vi "FPGAController_v4.vi"() -> ()   [LabVIEW 2013]
uses:
  <vilib>/rvi/interface/nirviOpenFPGA/nirviOpenFPGA.xnode
  <vilib>/rvi/interface/nirviMethod/nirviMethod.xnode
  <vilib>/rvi/interface/nirviReadWriteControl/nirviReadWriteControl.xnode
  <vilib>/rvi/interface/nirviCloseFPGA/nirviCloseFPGA.xnode
  <vilib>/addons/database/NI_Database_API.lvlib
  <vilib>/addons/database/Recordset.llb/Rec Fetch Recordset Data (R).vi
  <vilib>/addons/database/Connection.llb/Conn Execute.vi
  <vilib>/addons/database/_DB Variant To Data/Database Variant To Data.xnode
  <vilib>/addons/database/Recordset.llb/Rec Destroy - Connection.vi
  <vilib>/Utility/miscctls.llb/LVPointTypeDef.ctl
  <userlib>/Accelerator/User Interface/Executables/FPGAController_v4/data/correlationwithf_FPGATarget_FPGAcode60214_dpdmgs7o1BA.lvbitx
  <userlib>/_OpenG.lib/file/file.llb/Strip Path Extension - Path__ogtk.vi
  <userlib>/_OpenG.lib/comparison/comparison.llb/Boolean Changed__ogtk.vi
  <userlib>/_OpenG.lib/comparison/comparison.llb/DBL Changed__ogtk.vi
  <vilib>/rvi/errors/niLvFpgaMergeErrorWithErrorCode.vi
  <vilib>/FPGAPlugInAG/PXI-7954R/niLvFpga_Open_PXI-7954R.vi
panel:
  out "Time Betwee Shots":dbl
  out "Del Armed":bool
  in  "Lower Threshold":bool
  in  "Raise Threshold":bool
  out "Update Threshold":bool
  in  "Min. Time\nBetween Shots (s)":dbl
  in  "Rate Limiting":bool
  out "Armed":bool
  in  "Add Delay":bool
  in  "Delay Name":string
  in  "Delay Value":dbl=3.0 min=0.0
  in  "Delay Ring":dbl(ring)=3.15039 items=["Ablation Chamber"=6.45, "LEIL Chamber"=4.318, "Thid Detector"=3.15039, "Custom"=0.0]
  in  "Rearm Trigger":bool
  in  "One Shot Mode":bool
  out "Last Update:":timestamp
  out "Updating FPGA":bool
  out "Sensitivity":dbl
  out "error out":errorcluster
  out "Low Mass Limit":fxp<+,31,17>
  out "High Mass Limit":fxp<+,31,17>
  out "stopping":bool
  in  "Auto Threshold":bool
  out "Peletron (MV)":dbl=2.0
  out "High Mass (kg)":dbl=inf
  out "Low Mass (kg)":dbl
  out "High Charge Limit":i16
  out "Low Charge Limit":i16
  out "High velocity count":i32=210
  out "Low velocity count":i32=21000
  in  "stop":bool
  in  "Peak-Threshold Factor":dbl=2.0
  out "Low Charge Limit (fC)":dbl
  out "High Charge Limit (fC)":dbl=100.0
  out "High Velocity":dbl=100000.0
  out "Low Velocity":dbl=1000.0
  out "Filter 7 Peak":i32=7483
  out "Filter 6 Peak":i32=9863
  out "Filter 5 Peak":i32=13910
  out "Filter 4 Peak":i32=18191
  out "Filter 3 Peak":i32=46254
  out "Filter 2 Peak":i32=120664
  out "Filter 1 Peak":i32=295996
  in  "Filter7 Threshold":i32=-21165
  in  "Filter6 Threshold":i32=-29358
  in  "Filter5 Threshold":i32=-41730
  in  "Filter4 Threshold":i32=-54306
  in  "Filter3 Threshold":i32=-138762
  in  "Filter2 Threshold":i32=-361992
  in  "Filter1 Threshold":i32=-887988
  in  "Zero Peak Values":bool
  in  "Assign Threshold":bool
  in  "Run Mode":bool
  # "Settings"
  # "Dubugging"
  # "Independent Variable"
  # "Low Vel."
  # "High Vel."
  # "Low Q (fC)"
  # "High Q (fC)"
  # "Plate Control While Loop Counter"
  # "Low Mass (kg)"
  # "High Mass (kg)"
  # "Sens. (V/pC)"
  # "Peletron (MV)"
  # "Current Value of Running Average"
  # "Peak Threshold Factor"
  # "Delay Trigger"
  # "Dist. from 2nd Det. (m)"
  # "Name"
  # "Peak Values"
  # "Peak 1"
  # "Peak 2"
  # "Peak 3"
  # "Peak 4"
  # "Peak 5"
  # "Peak 6"
  # "Peak 7"
  # "Thresholds"
  # "Threshold 1"
  # "Threshold 2"
  # "Threshold 3"
  # "Threshold 4"
  # "Threshold 5"
  # "Threshold 6"
  # "Threshold 7"
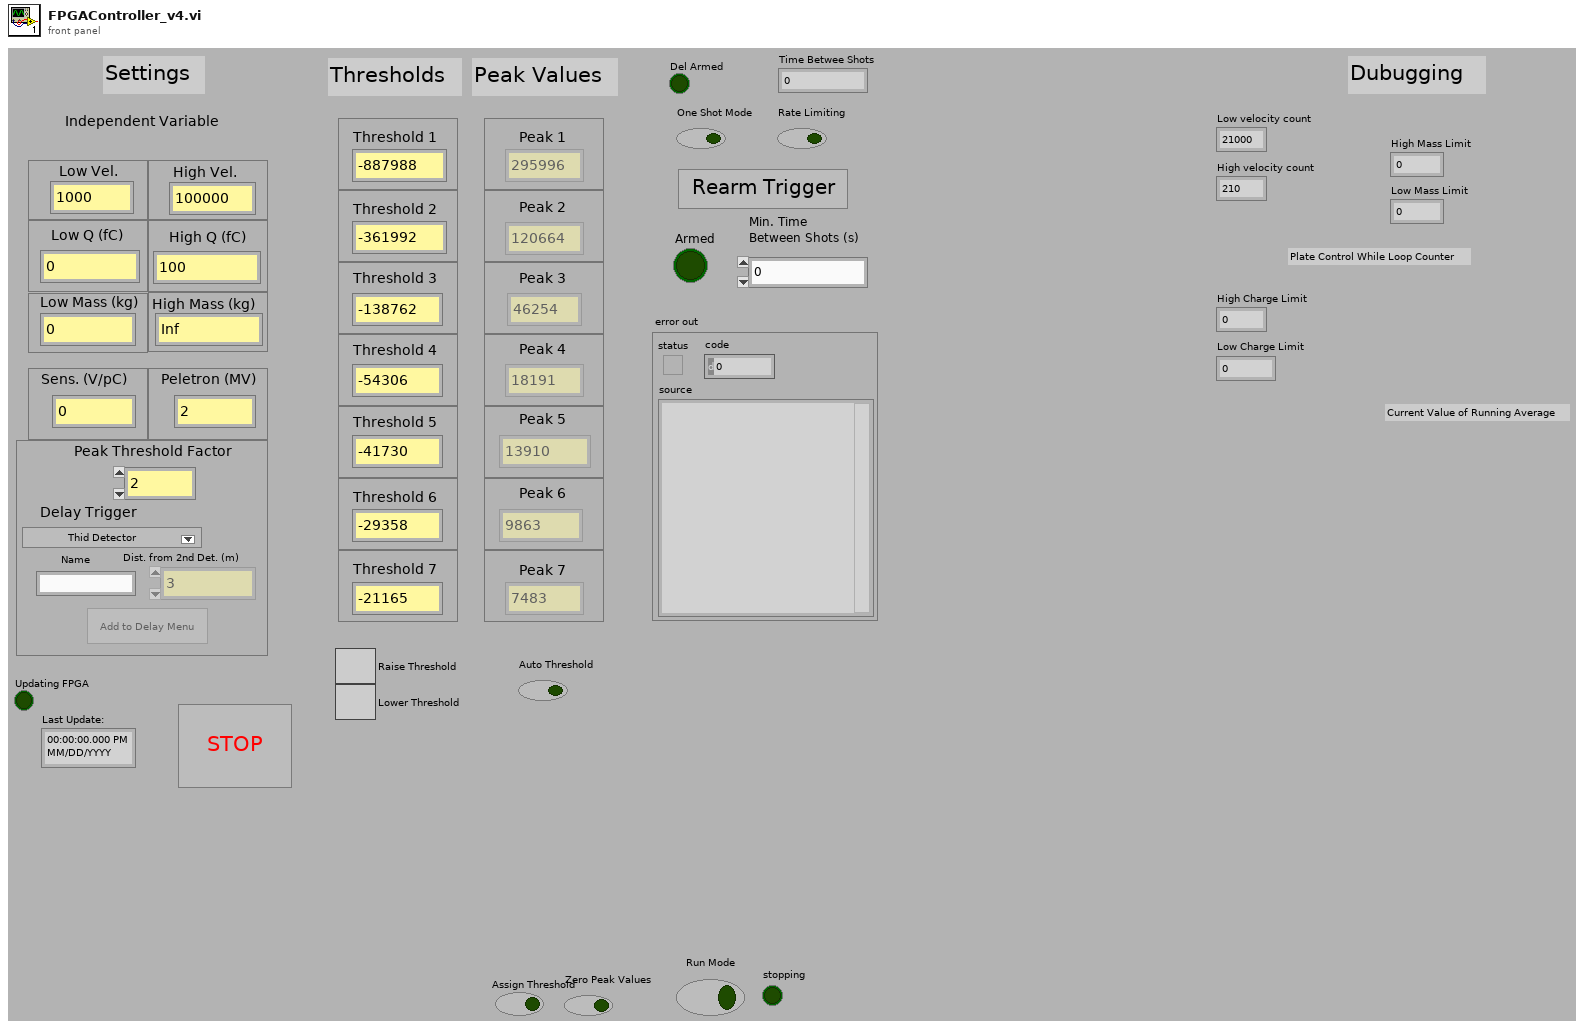
[diagram p1: front panel]
types:
  T1 = typedef "LVPointTypeDef.ctl" = cluster{"Horizontal":i16, "Vertical":i16}
  T2 = enum8{"Enabled", "Disabled", "Disabled and Grayed Out"}
  T3 = typedef "NI_Database_API.lvlib/Conn ObjectReference.ctl" = refnum<k1>
  T4 = cluster{"Filter 1 Peak":i32, "Filter 2 Peak":i32, "Filter 3 Peak":i32, "Filter 4 Peak":i32, "Filter 5 Peak":i32, "Filter 6 Peak":i32, "Filter 7 Peak":i32}
  T5 = typedef "NI_Database_API.lvlib/Rec ObjectReference.ctl" = refnum<k1>
  T6 = typedef "LVStringsAndValuesArrayTypeDef_DBL.ctl" = cluster{"String":string, "Value":dbl}[]
  T7 = cluster{"Numeric":dbl, "Numeric":dbl, "Numeric":dbl, "Numeric":dbl, "Numeric":dbl, "Numeric":dbl, dbl, dbl, "Value":dbl, fxp<+,16,7>, bool}
  T8 = cluster{"Low Velocity Count":i32, "High Velocity Count":i32, "Low Charge Limit (ADC ticks)":i16, "High Charge Limit (ADC ticks)":i16, "Low Mass (ADC*cycle^2)":i64, "High Mass (ADC*cycle^2)":i64, "Mult":fxp<+,16,7>, "Mult Use?":bool}
  T9 = cluster{"Filter 1 Detector 3 Correlation":void, "Filter 2 Detector 3 Correlation":void, "Filter 3 Detector 3 Correlation":void, "Filter 4 Detector 3 Correlation":void, "Filter 5 Detector 3 Correlation":void, "Filter 6 Detector 3 Correlation":void, "Filter 7 Detector 3 Correlation":void}
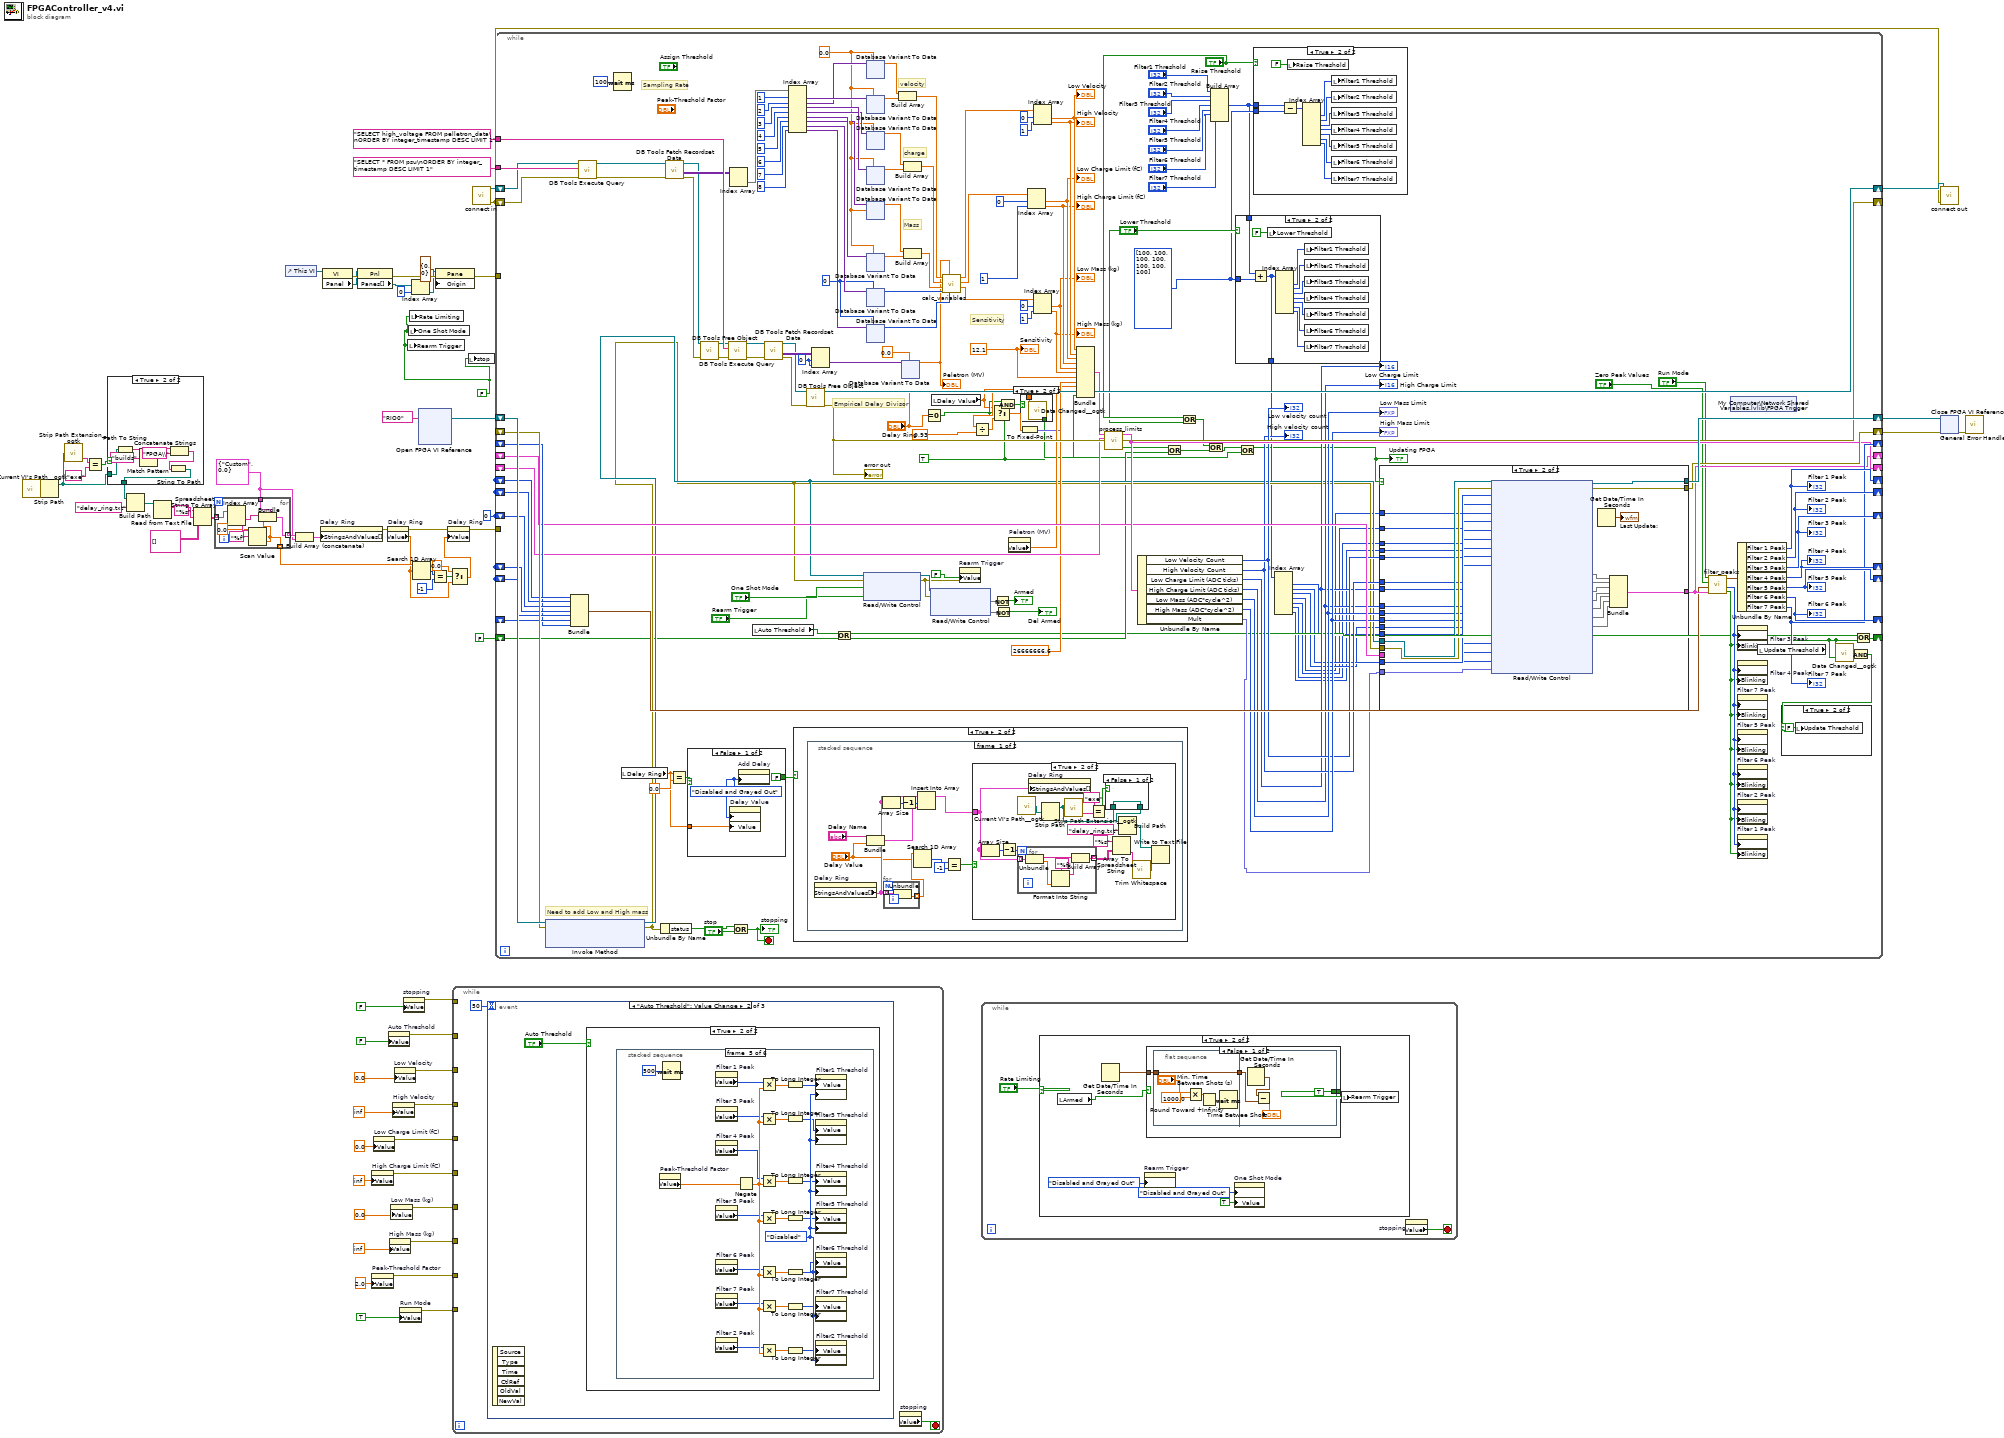
[diagram p0: block diagram]
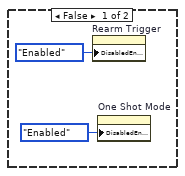
[diagram p3: hidden frame]
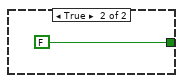
[diagram p4: hidden frame]
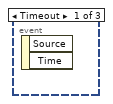
[diagram p5: hidden frame]
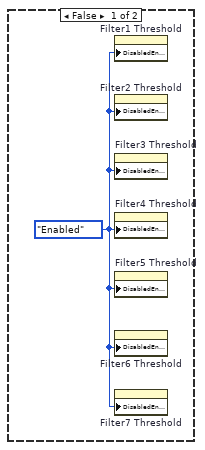
[diagram p6: hidden frame]
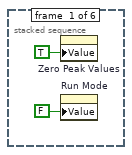
[diagram p7: hidden frame]
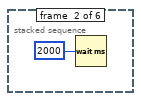
[diagram p8: hidden frame]
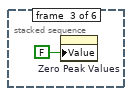
[diagram p9: hidden frame]
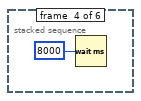
[diagram p10: hidden frame]
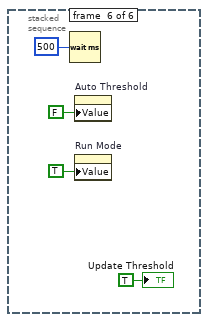
[diagram p11: hidden frame]
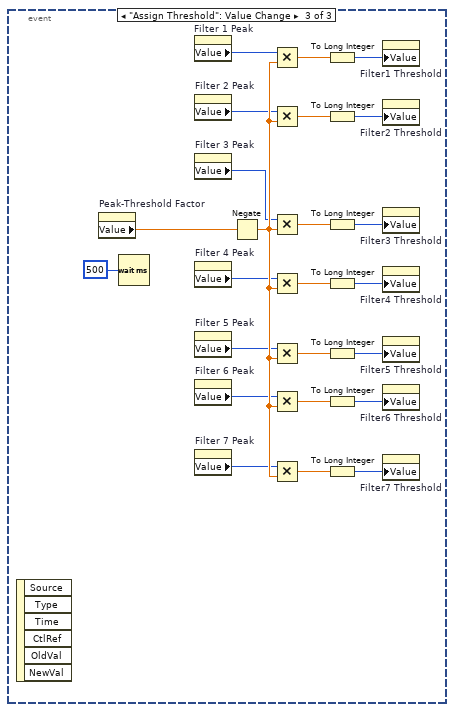
[diagram p12: hidden frame]
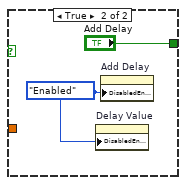
[diagram p17: hidden frame]
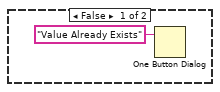
[diagram p19: hidden frame]
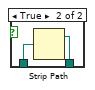
[diagram p20: hidden frame]
diagram:
  w17 = cluster{"String":string, "Value":dbl} {"String"="Custom", "Value"=0.0}
  w27 = FALSE
  w66 = 0
  n1 = call <userlib>:"Current VI's Path__ogtk.vi"() -> ("Current VI's Path (+ Relative)"=w26:path)  [unwired: 1 in]
  n2 = Strip Path(path=w26) -> (stripped path=w12:path)  [unwired: 1 out]
  n3 = call-poly <userlib>:"Strip Path Extension__ogtk.vi"("path"=w12) -> ("extension"=w16:string)  [unwired: 1 out]
  n4 = Equal?(x=w16, y="exe") -> (x = y?=w13:bool)
  n5 = case shown="True" w13 {
    tunnel: w12 -> [w68 w75]
    tunnel: [w68 w69] -> w11
    frame False {
    }
    frame True {
      n6 = Path To String(path=w75) -> (string=w74:string)
      n7 = Match Pattern(string=w74, regular expression="builds") -> (before substring=w72:string)  [unwired: 1 in, 3 out]
      n8 = Concatenate Strings(w72, "FPGA\\" ("string")) -> (w70:string)
      n9 = String To Path(string=w70) -> (path=w69:path)
    }
  }
  n10 = Build Path(base path=w11, name or relative path="delay_ring.txt") -> (appended path=w14:path)
  n11 = Read from Text File(file (use dialog)=w14) -> (text=w24:string)  [unwired: 3 in, 3 out]
  n12 = Spreadsheet String To Array(format string="%s", spreadsheet string=w24, array type (2D Dbl)=string[][] []) -> (array=w21:string[][])  [unwired: 1 in]
  n13 = for {
    tunnel: w21 -> [w83] mode=indexing
    tunnel: w17 -> [w81]
    tunnel: [w77] -> w18 mode=indexing
    tunnel: [w76] -> w10 mode=indexing
    n14 = Index Array(array=w83) -> (element #1=w82:string, element #2=w80:string)  [unwired: 2 in]
    n15 = Scan Value(string=w80, format string="%f", default (0 dbl)=0.0) -> (value=w76:dbl)  [unwired: 1 out]
    n16 = Bundle(cluster=w81, "String"=w82, "Value"=w76) -> (w77:cluster{"String":string, "Value":dbl})
  }
  n17 = control-ref of="This VI"() -> (w38:refnum<vi>)
  n18 = Build Array (concatenate)(w18, w17) -> (w20:cluster{"String":string, "Value":dbl}[])
  n19 = property on="Delay Ring" class="Ring (strict)"("StringsAndValues[]"=w20) -> (error out=w19:errorcluster)  [unwired: 2 in, 1 out]
  n20 = property class="VI"(reference=w38) -> (error out=w37:errorcluster, "Panel"=w36:refnum<vi>)  [unwired: 1 in, 1 out]
  n21 = property class="Pnl"(reference=w36, error in=w37) -> (error out=w35:errorcluster, "Panes[]"=w34:refnum<vi>[])  [unwired: 1 out]
  n22 = property on="High Charge Limit (fC)" class="DigNum (strict)"("Value"=inf ("High Charge Limit (fC)")) -> (error out=w53:errorcluster)  [unwired: 2 in, 1 out]
  n23 = property on="Peak-Threshold Factor" class="DigNum (strict)"("Value"=2.0 ("Peak-Threshold Factor")) -> (error out=w47:errorcluster)  [unwired: 2 in, 1 out]
  n24 = property on="Low Charge Limit (fC)" class="DigNum (strict)"("Value"=0.0 ("Low Charge Limit (fC)")) -> (error out=w55:errorcluster)  [unwired: 2 in, 1 out]
  n25 = property on="Delay Ring" class="Ring (strict)"(error in=w19) -> (error out=w9:errorcluster, "Value"=w3:dbl)  [unwired: 1 in, 1 out]
  n26 = property on="Auto Threshold" class="Bool (strict)"("Value"=FALSE ("Auto Threshold")) -> (error out=w61:errorcluster)  [unwired: 2 in, 1 out]
  n27 = property on="High Mass (kg)" class="DigNum (strict)"("Value"=inf ("High Mass (kg)")) -> (error out=w49:errorcluster)  [unwired: 2 in, 1 out]
  n28 = property on="Low Mass (kg)" class="DigNum (strict)"("Value"=0.0 ("Low Mass (kg)")) -> (error out=w51:errorcluster)  [unwired: 2 in, 1 out]
  n29 = property on="High Velocity" class="DigNum (strict)"("Value"=inf ("High Velocity")) -> (error out=w57:errorcluster)  [unwired: 2 in, 1 out]
  n30 = property on="Low Velocity" class="DigNum (strict)"("Value"=0.0 ("Low Velocity")) -> (error out=w59:errorcluster)  [unwired: 2 in, 1 out]
  n31 = property on="Run Mode" class="Bool (strict)"("Value"=TRUE ("Run Mode")) -> (error out=w45:errorcluster)  [unwired: 2 in, 1 out]
  n32 = property on="stopping" class="Bool (strict)"("Value"=FALSE ("stopping")) -> (error out=w63:errorcluster)  [unwired: 2 in, 1 out]
  n33 = local write "Rearm Trigger"(w27) -> ()
  n34 = local write "One Shot Mode"(w27) -> ()
  n35 = local write "Rate Limiting"(w27) -> ()
  n36 = Index Array(array=w34, index=0) -> (element=w32:refnum<vi>)
  n37 = Search 1D Array(1D array=w10, element=w3) -> (index of element=w7:i32)  [unwired: 1 in]
  n38 = xnode "Open FPGA VI Reference"("resource name"=tag "RIO0") -> ("FPGA VI Reference Out"=w29:refnum<k20>)  [unwired: 1 in, 1 out]
  n39 = Equal?(x=w7, y=-1) -> (x = y?=w5:bool)
  n40 = property class="Pane"(reference=w32, error in=w35, "Origin"=T1 {"Horizontal"=0, "Vertical"=0}) -> (error out=w30:errorcluster)  [unwired: 1 out]
  n41 = Select(t=0.0, s=w5, f=w3) -> (s? t:f=w4:dbl)
  n42 = property on="Delay Ring" class="Ring (strict)"(error in=w9, "Value"=w4) -> (error out=w8:errorcluster)  [unwired: 1 in, 1 out]
  n43 = while {
    tunnel: w63 -> [_]
    tunnel: w61 -> [_]
    tunnel: w59 -> [_]
    tunnel: w57 -> [_]
    tunnel: w55 -> [_]
    tunnel: w53 -> [_]
    tunnel: w51 -> [_]
    tunnel: w49 -> [_]
    tunnel: w47 -> [_]
    tunnel: w45 -> [_]
    stop <- w85 stop-if-true
    n44 = event shown="[1] \"Auto Threshold\": Value Change" {
      selector: _ -> [_ _ _]
      dyn-events: _ -> [_ _ _]
      timeout: 50 -> [_ _ _]
      event Timeout {
        n45 = event-data() -> ()  [unwired: 1 in, 2 out]
      }
      event "Auto Threshold": Value Change {
        n46 = event-data() -> ()  [unwired: 1 in, 6 out]
        n47 = case shown="True" "Auto Threshold" {
          frame False {
            w87 = T2."Enabled" ("Disabled")
            n48 = property on="Filter1 Threshold" class="DigNum (strict)"("DisabledEnum"=w87) -> ()  [unwired: 2 in, 2 out]
            n49 = property on="Filter2 Threshold" class="DigNum (strict)"("DisabledEnum"=w87) -> ()  [unwired: 2 in, 2 out]
            n50 = property on="Filter3 Threshold" class="DigNum (strict)"("DisabledEnum"=w87) -> ()  [unwired: 2 in, 2 out]
            n51 = property on="Filter4 Threshold" class="DigNum (strict)"("DisabledEnum"=w87) -> ()  [unwired: 2 in, 2 out]
            n52 = property on="Filter5 Threshold" class="DigNum (strict)"("DisabledEnum"=w87) -> ()  [unwired: 2 in, 2 out]
            n53 = property on="Filter6 Threshold" class="DigNum (strict)"("DisabledEnum"=w87) -> ()  [unwired: 2 in, 2 out]
            n54 = property on="Filter7 Threshold" class="DigNum (strict)"("DisabledEnum"=w87) -> ()  [unwired: 2 in, 2 out]
          }
          frame True {
            n55 = stacked-sequence {
              frame #0 {
                n56 = property on="Zero Peak Values" class="Bool (strict)"("Value"=TRUE ("Zero Peak Values")) -> ()  [unwired: 2 in, 2 out]
                n57 = property on="Run Mode" class="Bool (strict)"("Value"=FALSE ("Run Mode")) -> ()  [unwired: 2 in, 2 out]
              }
              frame #1 {
                n58 = Wait (ms)(milliseconds to wait=u32 2000) -> ()  [unwired: 1 out]
              }
              frame #2 {
                n59 = property on="Zero Peak Values" class="Bool (strict)"("Value"=FALSE ("Zero Peak Values")) -> ()  [unwired: 2 in, 2 out]
              }
              frame #3 {
                n60 = Wait (ms)(milliseconds to wait=u32 8000) -> ()  [unwired: 1 out]
              }
              frame #4 {
                w117 = T2."Disabled" ("Disabled")
                n61 = property on="Peak-Threshold Factor" class="DigNum (strict)"() -> ("Value"=w102:dbl)  [unwired: 2 in, 2 out]
                n62 = Wait (ms)(milliseconds to wait=u32 500) -> ()  [unwired: 1 out]
                n63 = property on="Filter 1 Peak" class="DigNum (strict)"() -> ("Value"=w100:i32)  [unwired: 2 in, 2 out]
                n64 = property on="Filter 3 Peak" class="DigNum (strict)"() -> ("Value"=w98:i32)  [unwired: 2 in, 2 out]
                n65 = property on="Filter 4 Peak" class="DigNum (strict)"() -> ("Value"=w97:i32)  [unwired: 2 in, 2 out]
                n66 = property on="Filter 5 Peak" class="DigNum (strict)"() -> ("Value"=w96:i32)  [unwired: 2 in, 2 out]
                n67 = property on="Filter 6 Peak" class="DigNum (strict)"() -> ("Value"=w95:i32)  [unwired: 2 in, 2 out]
                n68 = property on="Filter 7 Peak" class="DigNum (strict)"() -> ("Value"=w94:i32)  [unwired: 2 in, 2 out]
                n69 = property on="Filter 2 Peak" class="DigNum (strict)"() -> ("Value"=w99:i32)  [unwired: 2 in, 2 out]
                n70 = Negate(x=w102) -> (-x=w101:dbl)
                n71 = Multiply(x=w100, y=w101) -> (x*y=w116:dbl)
                n72 = Multiply(x=w98, y=w101) -> (x*y=w112:dbl)
                n73 = Multiply(x=w97, y=w101) -> (x*y=w110:dbl)
                n74 = Multiply(x=w96, y=w101) -> (x*y=w108:dbl)
                n75 = Multiply(x=w95, y=w101) -> (x*y=w106:dbl)
                n76 = Multiply(x=w94, y=w101) -> (x*y=w104:dbl)
                n77 = Multiply(x=w99, y=w101) -> (x*y=w114:dbl)
                n78 = To Long Integer(number=w116) -> (32bit integer=w115:i32)
                n79 = To Long Integer(number=w112) -> (32bit integer=w111:i32)
                n80 = To Long Integer(number=w110) -> (32bit integer=w109:i32)
                n81 = To Long Integer(number=w108) -> (32bit integer=w107:i32)
                n82 = To Long Integer(number=w106) -> (32bit integer=w105:i32)
                n83 = To Long Integer(number=w104) -> (32bit integer=w103:i32)
                n84 = To Long Integer(number=w114) -> (32bit integer=w113:i32)
                n85 = property on="Filter1 Threshold" class="DigNum (strict)"("Value"=w115, "DisabledEnum"=w117) -> ()  [unwired: 2 in, 2 out]
                n86 = property on="Filter3 Threshold" class="DigNum (strict)"("Value"=w111, "DisabledEnum"=w117) -> ()  [unwired: 2 in, 2 out]
                n87 = property on="Filter4 Threshold" class="DigNum (strict)"("Value"=w109, "DisabledEnum"=w117) -> ()  [unwired: 2 in, 2 out]
                n88 = property on="Filter5 Threshold" class="DigNum (strict)"("Value"=w107, "DisabledEnum"=w117) -> ()  [unwired: 2 in, 2 out]
                n89 = property on="Filter6 Threshold" class="DigNum (strict)"("Value"=w105, "DisabledEnum"=w117) -> ()  [unwired: 2 in, 2 out]
                n90 = property on="Filter7 Threshold" class="DigNum (strict)"("Value"=w103, "DisabledEnum"=w117) -> ()  [unwired: 2 in, 2 out]
                n91 = property on="Filter2 Threshold" class="DigNum (strict)"("Value"=w113, "DisabledEnum"=w117) -> ()  [unwired: 2 in, 2 out]
              }
              frame #5 {
                n92 = Wait (ms)(milliseconds to wait=u32 500) -> ()  [unwired: 1 out]
                n93 = property on="Auto Threshold" class="Bool (strict)"("Value"=FALSE ("Auto Threshold")) -> ()  [unwired: 2 in, 2 out]
                n94 = property on="Run Mode" class="Bool (strict)"("Value"=TRUE ("Run Mode")) -> ()  [unwired: 2 in, 2 out]
                "Update Threshold" <- TRUE ("Update Threshold")
              }
            }
          }
        }
      }
      event "Assign Threshold": Value Change {
        n95 = event-data() -> ()  [unwired: 1 in, 6 out]
        n96 = property on="Peak-Threshold Factor" class="DigNum (strict)"() -> ("Value"=w136:dbl)  [unwired: 2 in, 2 out]
        n97 = Wait (ms)(milliseconds to wait=u32 500) -> ()  [unwired: 1 out]
        n98 = property on="Filter 1 Peak" class="DigNum (strict)"() -> ("Value"=w135:i32)  [unwired: 2 in, 2 out]
        n99 = property on="Filter 2 Peak" class="DigNum (strict)"() -> ("Value"=w134:i32)  [unwired: 2 in, 2 out]
        n100 = property on="Filter 3 Peak" class="DigNum (strict)"() -> ("Value"=w133:i32)  [unwired: 2 in, 2 out]
        n101 = property on="Filter 4 Peak" class="DigNum (strict)"() -> ("Value"=w132:i32)  [unwired: 2 in, 2 out]
        n102 = property on="Filter 5 Peak" class="DigNum (strict)"() -> ("Value"=w131:i32)  [unwired: 2 in, 2 out]
        n103 = property on="Filter 6 Peak" class="DigNum (strict)"() -> ("Value"=w130:i32)  [unwired: 2 in, 2 out]
        n104 = property on="Filter 7 Peak" class="DigNum (strict)"() -> ("Value"=w129:i32)  [unwired: 2 in, 2 out]
        n105 = Negate(x=w136) -> (-x=w138:dbl)
        n106 = Multiply(x=w135, y=w138) -> (x*y=w145:dbl)
        n107 = Multiply(x=w134, y=w138) -> (x*y=w143:dbl)
        n108 = Multiply(x=w133, y=w138) -> (x*y=w142:dbl)
        n109 = Multiply(x=w132, y=w138) -> (x*y=w141:dbl)
        n110 = Multiply(x=w131, y=w138) -> (x*y=w140:dbl)
        n111 = Multiply(x=w130, y=w138) -> (x*y=w139:dbl)
        n112 = Multiply(x=w129, y=w138) -> (x*y=w144:dbl)
        n113 = To Long Integer(number=w145) -> (32bit integer=w128:i32)
        n114 = To Long Integer(number=w143) -> (32bit integer=w127:i32)
        n115 = To Long Integer(number=w142) -> (32bit integer=w126:i32)
        n116 = To Long Integer(number=w141) -> (32bit integer=w125:i32)
        n117 = To Long Integer(number=w140) -> (32bit integer=w124:i32)
        n118 = To Long Integer(number=w139) -> (32bit integer=w123:i32)
        n119 = To Long Integer(number=w144) -> (32bit integer=w122:i32)
        n120 = property on="Filter1 Threshold" class="DigNum (strict)"("Value"=w128) -> ()  [unwired: 2 in, 2 out]
        n121 = property on="Filter2 Threshold" class="DigNum (strict)"("Value"=w127) -> ()  [unwired: 2 in, 2 out]
        n122 = property on="Filter3 Threshold" class="DigNum (strict)"("Value"=w126) -> ()  [unwired: 2 in, 2 out]
        n123 = property on="Filter4 Threshold" class="DigNum (strict)"("Value"=w125) -> ()  [unwired: 2 in, 2 out]
        n124 = property on="Filter5 Threshold" class="DigNum (strict)"("Value"=w124) -> ()  [unwired: 2 in, 2 out]
        n125 = property on="Filter6 Threshold" class="DigNum (strict)"("Value"=w123) -> ()  [unwired: 2 in, 2 out]
        n126 = property on="Filter7 Threshold" class="DigNum (strict)"("Value"=w122) -> ()  [unwired: 2 in, 2 out]
      }
    }
    n127 = property on="stopping" class="Bool (strict)"() -> ("Value"=w85:bool)  [unwired: 2 in, 2 out]
  }
  n128 = local write "stop"(w27) -> ()
  n129 = call "connect in.vi"() -> ("error out"=w39:errorcluster, "Database Connection"=w40:T3)  [unwired: 7 in, 1 out]
  n130 = while {
    shift-right: [w307] -> w65
    shift-left: w29 -> [w311]
    shift-right: [w306] -> w64
    shift-left: _ -> [w310]
    shift-right: [w302] -> _
    shift-left: w66 -> [w295]
    shift-right: [w301] -> _
    shift-left: w66 -> [w294]
    shift-right: [w300] -> _
    shift-left: w66 -> [w293]
    shift-right: [w299] -> _
    shift-left: w66 -> [w292]
    shift-right: [w298] -> _
    shift-left: w66 -> [w291]
    shift-right: [w304] -> _
    shift-left: w66 -> [w297]
    shift-right: [w303] -> _
    shift-left: w66 -> [w296]
    tunnel: "SELECT * FROM psu\nORDER BY integer_timestamp DESC LIMIT 1" ("SQL query") -> [w290]
    tunnel: "SELECT high_voltage FROM pelletron_data\nORDER BY integer_timestamp DESC LIMIT 1" ("SQL query") -> [w289]
    shift-right: [w285] -> w41
    shift-left: w40 -> [w288]
    shift-right: [w286] -> _
    shift-left: w39 -> [w287]
    shift-right: [w284] -> _
    shift-left: _ -> [w283]
    shift-right: [w281] -> _
    shift-left: _ -> [w282]
    tunnel: w30 -> [_]
    tunnel: w8 -> [_]
    shift-right: [w185] -> _
    shift-left: FALSE -> [w188]
    stop <- w305 stop-if-true
    w147 = i32[] [100, 100, 100, 100, 100, 100, 100]
    w150 = TRUE
    w237 = 0 ("index (row)")
    w245 = i8 0
    w246 = 0.0
    w211 = 12.1
    # "charge"
    # "Empirical Delay Divisor"
    # "Mass"
    # "velocity"
    # "Sensitivity"
    # "Sampling Rate"
    # "Need to add Low and High mass"
    n131 = xnode "Invoke Method"("FPGA VI Reference In"=w311, "error in"=w310) -> ("FPGA VI Reference Out"=w205:refnum<k20>, "error out"=w204:errorcluster)  [unwired: 1 out]
    n132 = Bundle("Filter 1 Peak"=w297, "Filter 2 Peak"=w296, "Filter 3 Peak"=w295, "Filter 4 Peak"=w294, "Filter 5 Peak"=w293, "Filter 6 Peak"=w292, "Filter 7 Peak"=w291) -> (w277:T4)  [unwired: 1 in]
    n133 = call-poly <vilib>:"DB Tools Execute Query.vi"("error in (no error)"=w287, "SQL query"=w290, "connection reference"=w288) -> ("error out"=w265:errorcluster, "recordset reference"=w266:T5)  [unwired: 5 in]
    n134 = Wait (ms)(milliseconds to wait=u32 100) -> ()  [unwired: 1 out]
    n135 = local read "Delay Ring"() -> (w189:dbl)
    n136 = Unbundle By Name(w204) -> ("status"=w309:bool)
    n137 = call-poly <vilib>:"DB Tools Fetch Recordset Data.vi"("error in (no error)"=w265, "recordset reference"=w266) -> ("error out"=w243:errorcluster, "recordset data"=w256:variant[][], "recordset reference out"=w244:T5)  [unwired: 3 in]
    n138 = Equal?(x=w189, y=0.0) -> (x = y?=w190:bool)
    n139 = case shown="False" w190 {
      tunnel: [FALSE ("Add Delay") "Add Delay"] -> w208
      tunnel: w189 -> [w340 _]
      frame False {
        w341 = T2."Disabled and Grayed Out" ("Disabled")
        n140 = property on="Delay Value" class="DigNum (strict)"("DisabledEnum"=w341, "Value"=w340) -> ()  [unwired: 2 in, 2 out]
        n141 = property on="Add Delay" class="Bool (strict)"("DisabledEnum"=w341) -> ()  [unwired: 2 in, 2 out]
      }
      frame True {
        w342 = T2."Enabled" ("Disabled")
        n142 = property on="Delay Value" class="DigNum (strict)"("DisabledEnum"=w342) -> ()  [unwired: 2 in, 2 out]
        n143 = property on="Add Delay" class="Bool (strict)"("DisabledEnum"=w342) -> ()  [unwired: 2 in, 2 out]
      }
    }
    n144 = call-poly <vilib>:"DB Tools Free Object.vi"("error in (no error)"=w243, "recordset reference"=w244) -> ("error out"=w241:errorcluster, "connection reference"=w242:T3)  [unwired: 8 in]
    n145 = call-poly <vilib>:"DB Tools Execute Query.vi"("error in (no error)"=w241, "SQL query"=w289, "connection reference"=w242) -> ("error out"=w239:errorcluster, "recordset reference"=w240:T5)  [unwired: 5 in]
    n146 = Index Array(array=w256) -> (element=w255:variant[])  [unwired: 2 in]
    n147 = Or(x=w309, y="stop") -> (x .or. y?=w305:bool)
    "stopping" <- w305
    n148 = local read "Auto Threshold"() -> (w186:bool)
    n149 = call-poly <vilib>:"DB Tools Fetch Recordset Data.vi"("error in (no error)"=w239, "recordset reference"=w240) -> ("error out"=w212:errorcluster, "recordset data"=w238:variant[][], "recordset reference out"=w213:T5)  [unwired: 3 in]
    n150 = Index Array(array=w255, index #1=1 ("index"), index #2=2 ("index"), index #3=3 ("index"), index #4=4 ("index"), index #5=5 ("index"), index #6=6 ("index"), index #7=7 ("index"), index #8=8 ("index")) -> (element #1=w254:variant, element #2=w253:variant, element #3=w252:variant, element #4=w251:variant, element #5=w250:variant, element #6=w249:variant, element #7=w248:variant, element #8=w247:variant)
    n151 = case shown="True" w208 {
      frame False {
      }
      frame True {
        n152 = stacked-sequence {
          frame #0 {
            n153 = property on="Delay Ring" class="Ring (strict)"() -> ("StringsAndValues[]"=w346:T6)  [unwired: 2 in, 2 out]
            n154 = Bundle("Delay Name"="Delay Name", "Delay Value"="Delay Value") -> (w351:cluster{"Delay Name":string, "Delay Value":dbl})  [unwired: 1 in]
            n155 = Array Size(array=w346) -> (size(s)=w349:i32)
            n156 = for {
              tunnel: w346 -> [w356] mode=indexing
              tunnel: [w355] -> w345 mode=indexing
              n157 = Unbundle(w356) -> ("Value"=w355:dbl)  [unwired: 1 out]
            }
            n158 = Decrement(x=w349) -> (x-1=w348:i32)
            n159 = Search 1D Array(1D array=w345, element="Delay Value") -> (index of element=w353:i32)  [unwired: 1 in]
            n160 = Insert Into Array(array=w346, index=w348, new element=w351) -> (w350:T6)
            n161 = Equal?(x=w353, y=-1) -> (x = y?=w347:bool)
            n162 = case shown="True" w347 {
              tunnel: w350 -> [_ w365]
              frame False {
                n163 = One Button Dialog(message="Value Already Exists") -> ()  [unwired: 1 in, 1 out]
              }
              frame True {
                n164 = Array Size(array=w365) -> (size(s)=w367:i32)
                n165 = Decrement(x=w367) -> (x-1=w366:i32)
                n166 = call <userlib>:"Current VI's Path__ogtk.vi"() -> ("Current VI's Path (+ Relative)"=w371:path)  [unwired: 1 in]
                n167 = for {
                  N: w366 -> [_]
                  tunnel: w365 -> [w381] mode=indexing
                  tunnel: [w376] -> w368 mode=indexing
                  n168 = Unbundle(w381) -> ("String"=w377:string, "Value"=w380:dbl)
                  n169 = Format Into String(format string="%f", w380) -> (resulting string=w378:string)  [unwired: 2 in, 1 out]
                  n170 = Build Array(w377, w378) -> (w376:string[])
                }
                n171 = property on="Delay Ring" class="Ring (strict)"("StringsAndValues[]"=w365) -> ()  [unwired: 2 in, 2 out]
                n172 = Strip Path(path=w371) -> (stripped path=w359:path)  [unwired: 1 out]
                n173 = call-poly <userlib>:"Strip Path Extension__ogtk.vi"("path"=w359) -> ("extension"=w362:string)  [unwired: 1 out]
                n174 = Equal?(x="exe", y=w362) -> (x = y?=w360:bool)
                n175 = case shown="False" w360 {
                  tunnel: w359 -> [w373 w375]
                  tunnel: [w373 w374] -> w358
                  frame False {
                  }
                  frame True {
                    n176 = Strip Path(path=w375) -> (stripped path=w374:path)  [unwired: 1 out]
                  }
                }
                n177 = Array To Spreadsheet String(array=w368, 3:"%s" ("format string")) -> (spreadsheet string=w364:string)  [unwired: 1 in]
                n178 = Build Path(base path=w358, name or relative path="delay_ring.txt") -> (appended path=w369:path)
                n179 = call <vilib>:"Trim Whitespace.vi"("string"=w364) -> ("trimmed string"=w363:string)  [unwired: 1 in]
                n180 = Write to Text File(file (use dialog)=w369, text=w363) -> ()  [unwired: 2 in, 3 out]
              }
            }
          }
          frame #1 {
            n181 = property on="Add Delay" class="Bool (strict)"("Value"=FALSE ("Add Delay")) -> ()  [unwired: 2 in, 2 out]
          }
        }
      }
    }
    n182 = call-poly <vilib>:"DB Tools Free Object.vi"("error in (no error)"=w212, "recordset reference"=w213) -> ("error out"=w286:errorcluster, "connection reference"=w285:T3)  [unwired: 8 in]
    "error out" <- w286
    n183 = Index Array(array=w238, index (row)=w237, index (col)=w237) -> (element=w236:variant)
    n184 = Or(x=w186, y=w188) -> (x .or. y?=w187:bool)
    n185 = xnode "Read/Write Control"("FPGA VI Reference In"=w205, "error in"=w204, "One Shot"="One Shot Mode", "Reset One Shot"="Rearm Trigger") -> ("FPGA VI Reference Out"=w198:refnum<k20>, "error out"=w197:errorcluster)
    n186 = xnode "Database Variant To Data"("database variant"=w253, "type"=w246) -> ("data"=w161:dbl)  [unwired: 1 in, 1 out]
    n187 = xnode "Database Variant To Data"("database variant"=w254, "type"=w246) -> ("data"=w162:dbl)  [unwired: 1 in, 1 out]
    n188 = xnode "Database Variant To Data"("database variant"=w251, "type"=w246) -> ("data"=w160:dbl)  [unwired: 1 in, 1 out]
    n189 = xnode "Database Variant To Data"("database variant"=w252, "type"=w246) -> ("data"=w159:dbl)  [unwired: 1 in, 1 out]
    n190 = xnode "Database Variant To Data"("database variant"=w249, "type"=w246) -> ("data"=w158:dbl)  [unwired: 1 in, 1 out]
    n191 = xnode "Database Variant To Data"("database variant"=w250, "type"=w246) -> ("data"=w157:dbl)  [unwired: 1 in, 1 out]
    n192 = xnode "Database Variant To Data"("database variant"=w248, "type"=w245) -> ("data"=w230:i8)  [unwired: 1 in, 1 out]
    n193 = xnode "Database Variant To Data"("database variant"=w247, "type"=w245) -> ("data"=w229:i8)  [unwired: 1 in, 1 out]
    n194 = Build Array(w161, w162) -> (w233:dbl[])
    n195 = xnode "Database Variant To Data"("database variant"=w236, "type"=0.0) -> ("data"=w156:dbl)  [unwired: 1 in, 1 out]
    "Peletron (MV)" <- w156
    n196 = Build Array(w160, w159) -> (w232:dbl[])
    n197 = Build Array(w158, w157) -> (w231:dbl[])
    n198 = Equal To 0?(x="Delay Ring") -> (x = 0?=w155:bool)
    n199 = xnode "Read/Write Control"("FPGA VI Reference In"=w198, "error in"=w197) -> ("Not Armed?"=w196, "Del Not Armed?"=w149)  [unwired: 2 out]
    n200 = local read "Delay Value"() -> (w154:dbl)
    n201 = call "calc_variables.vi"("var2"=w229, "Peletron"=w156, "var1"=w230, "Mass"=w231, "Charge"=w232, "Velocity"=w233) -> ("Mass out"=w222:dbl[], "Charge out"=w225:dbl[], "Velocity out"=w228:dbl[])  [unwired: 3 in]
    n202 = property on="Rearm Trigger" class="Bool (strict)"(error in=w197, "Value"=FALSE ("Rearm Trigger")) -> ()  [unwired: 1 in, 2 out]
    n203 = Divide(x="Delay Ring", y=0.93) -> (x/y=w194:dbl)
    n204 = Select(t=w154, s=w155, f=w194) -> (s? t:f=w193:dbl)
    n205 = Not(x=w196) -> (.not. x?=→"Armed":bool)
    n206 = Not(x=w149) -> (.not. x?=→"Del Armed":bool)
    n207 = And(x=w155, y=w150) -> (x .and. y?=w151:bool)
    n208 = property on="Peletron (MV)" class="DigNum (strict)"() -> ("Value"=w234:dbl)  [unwired: 2 in, 2 out]
    n209 = case shown="True" w151 {
      selector: w151 -> [w312 _]
      tunnel: w154 -> [_ w314]
      tunnel: [w312 w313] -> w152
      frame False {
      }
      frame True {
        n210 = call-poly <userlib>:"Data Changed__ogtk.vi"("DBL"=w314) -> ("Changed"=w313:bool)
      }
    }
    n211 = To Fixed-Point(number=w193) -> (fixed-point=w207:fxp<+,16,7>)  [unwired: 1 in]
    n212 = Index Array(array=w225, index #1=0 ("index"), index #2=1 ("index")) -> (element #1=w217:dbl, element #2=w216:dbl)
    "High Charge Limit (fC)" <- w216
    "Low Charge Limit (fC)" <- w217
    n213 = Index Array(array=w228, index #1=0 ("index"), index #2=1 ("index")) -> (element #1=w219:dbl, element #2=w218:dbl)
    "High Velocity" <- w218
    "Low Velocity" <- w219
    n214 = Index Array(array=w222, index #1=0 ("index"), index #2=1 ("index")) -> (element #1=w215:dbl, element #2=w214:dbl)
    "Low Mass (kg)" <- w215
    "High Mass (kg)" <- w214
    n215 = Bundle("Numeric"=w219, "Numeric"=w218, "Numeric"=w217, "Numeric"=w216, "Numeric"=w215, "Numeric"=w214, w211, 26666666.6, "Value"=w234, w207, w150) -> (w276:T7)  [unwired: 1 in]
    n216 = call "process_limits.vi"("old output cluster"=w283, "Input cluster"=w276) -> ("Update FPGA"=w210:bool, "output cluster"=w284:T8)  [unwired: 8 in]
    n217 = Unbundle By Name(w284) -> ("Low Velocity Count"=w272:i32, "High Velocity Count"=w271:i32, "Low Charge Limit (ADC ticks)"=w269:i16, "High Charge Limit (ADC ticks)"=w270:i16, "Low Mass (ADC*cycle^2)"=w274:i64, "High Mass (ADC*cycle^2)"=w275:i64, "Mult"=w206:fxp<+,16,7>)
    "Low velocity count" <- w272
    "High velocity count" <- w271
    "High Charge Limit" <- w270
    "Low Charge Limit" <- w269
    "High Mass Limit" <- w275
    "Low Mass Limit" <- w274
    n218 = Or(x=w210, y=w187) -> (x .or. y?=w192:bool)
    n219 = Or(x="Raise Threshold", y="Lower Threshold") -> (x .or. y?=w163:bool)
    n220 = Or(x=w163, y=w192) -> (x .or. y?=w164:bool)
    n221 = Build Array("Filter1 Threshold", "Filter2 Threshold", "Filter3 Threshold", "Filter4 Threshold", "Filter5 Threshold", "Filter6 Threshold", "Filter7 Threshold") -> (w146:i32[])
    n222 = case shown="True" "Lower Threshold" {
      tunnel: w146 -> [w315 w326]
      tunnel: w147 -> [_ w325]
      tunnel: [w315 w316] -> w177
      frame False {
      }
      frame True {
        n223 = Add(x=w326, y=w325) -> (x+y=w316:i32[])
        n224 = local write "Lower Threshold"(FALSE ("Lower Threshold")) -> ()
        n225 = Index Array(array=w316) -> (element #1=w323:i32, element #2=w322:i32, element #3=w321:i32, element #4=w320:i32, element #5=w319:i32, element #6=w318:i32, element #7=w317:i32)  [unwired: 7 in]
        n226 = local write "Filter1 Threshold"(w323) -> ()
        n227 = local write "Filter2 Threshold"(w322) -> ()
        n228 = local write "Filter3 Threshold"(w321) -> ()
        n229 = local write "Filter4 Threshold"(w320) -> ()
        n230 = local write "Filter5 Threshold"(w319) -> ()
        n231 = local write "Filter6 Threshold"(w318) -> ()
        n232 = local write "Filter7 Threshold"(w317) -> ()
      }
    }
    n233 = Or(x=w164, y=w152) -> (x .or. y?=w153:bool)
    "Updating FPGA" <- w153
    n234 = case shown="True" "Raise Threshold" {
      tunnel: w146 -> [_ w337]
      tunnel: w147 -> [_ w327]
      frame False {
      }
      frame True {
        n235 = Subtract(x=w337, y=w327) -> (x-y=w328:i32[])
        n236 = local write "Raise Threshold"(FALSE ("Raise Threshold")) -> ()
        n237 = Index Array(array=w328) -> (element #1=w335:i32, element #2=w334:i32, element #3=w333:i32, element #4=w332:i32, element #5=w331:i32, element #6=w330:i32, element #7=w329:i32)  [unwired: 7 in]
        n238 = local write "Filter1 Threshold"(w335) -> ()
        n239 = local write "Filter2 Threshold"(w334) -> ()
        n240 = local write "Filter3 Threshold"(w333) -> ()
        n241 = local write "Filter4 Threshold"(w332) -> ()
        n242 = local write "Filter5 Threshold"(w331) -> ()
        n243 = local write "Filter6 Threshold"(w330) -> ()
        n244 = local write "Filter7 Threshold"(w329) -> ()
      }
    }
    n245 = Index Array(array=w177) -> (element #1=w180:i32, element #2=w178:i32, element #3=w175:i32, element #4=w173:i32, element #5=w171:i32, element #6=w169:i32, element #7=w167:i32)  [unwired: 7 in]
    n246 = case shown="True" w153 {
      tunnel: w205 -> [w384 w412]
      tunnel: w204 -> [w385 w411]
      tunnel: [w384 w410] -> w307
      tunnel: [w385 w409] -> w306
      tunnel: w180 -> [_ w408]
      tunnel: w178 -> [_ w407]
      tunnel: w175 -> [_ w406]
      tunnel: w173 -> [_ w405]
      tunnel: w171 -> [_ w404]
      tunnel: w169 -> [_ w403]
      tunnel: w167 -> [_ w402]
      tunnel: [w383 w388] -> w281
      tunnel: w275 -> [_ w394]
      tunnel: w274 -> [_ w393]
      tunnel: w272 -> [_ w392]
      tunnel: w271 -> [_ w391]
      tunnel: w270 -> [_ w390]
      tunnel: w269 -> [_ w389]
      tunnel: w282 -> [w383 _]
      tunnel: w206 -> [_ w386]
      frame False {
      }
      frame True {
        n247 = xnode "Read/Write Control"("FPGA VI Reference In"=w412, "error in"=w411, "Low Velocity Count"=w392, "High Velocity Count"=w391, "Filter 1 threshold"=w408, "Filter 2 threshold"=w407, "Filter 3 threshold"=w406, "Filter 4 threshold"=w405, "Filter 5 threshold"=w404, "Filter 6 threshold"=w403, "Filter 7 threshold"=w402, "High Charge Limit"=w390, "Low Charge Limit"=w389, "High Mass Limit"=w394, "Low Mass Limit"=w393, "Mult1"=w386) -> ("FPGA VI Reference Out"=w410:refnum<k20>, "error out"=w409:errorcluster, "Filter 1 Detector 3 Correlation"=w401, "Filter 2 Detector 3 Correlation"=w400, "Filter 3 Detector 3 Correlation"=w399, "Filter 4 Detector 3 Correlation"=w398, "Filter 5 Detector 3 Correlation"=w397, "Filter 6 Detector 3 Correlation"=w396, "Filter 7 Detector 3 Correlation"=w395)
        n248 = Get Date/Time In Seconds() -> (seconds since 1Jan1904=→"Last Update:":timestamp)
        n249 = Bundle("Filter 1 Detector 3 Correlation"=w401, "Filter 2 Detector 3 Correlation"=w400, "Filter 3 Detector 3 Correlation"=w399, "Filter 4 Detector 3 Correlation"=w398, "Filter 5 Detector 3 Correlation"=w397, "Filter 6 Detector 3 Correlation"=w396, "Filter 7 Detector 3 Correlation"=w395) -> (w388:T9)  [unwired: 1 in]
      }
    }
    n250 = call "filter_peaks.vi"("Correlation cluster"=w281, "Filter peak cluster"=w277, "Zero out"="Zero Peak Values", "Run Mode"="Run Mode") -> ("Blinking"=w268:bool, "status"=w273:T2, "Filter peak output"=w278:T4)  [unwired: 5 in]
    n251 = shared-variable "My Computer\\Network Shared Variables.lvlib\\FPGA Trigger"() -> ()  [unwired: 1 in, 2 out]
    n252 = Unbundle By Name(w278) -> ("Filter 1 Peak"=w304:i32, "Filter 2 Peak"=w303:i32, "Filter 3 Peak"=w302:i32, "Filter 4 Peak"=w301:i32, "Filter 5 Peak"=w300:i32, "Filter 6 Peak"=w299:i32, "Filter 7 Peak"=w298:i32)
    "Filter 1 Peak" <- w304
    "Filter 2 Peak" <- w303
    "Filter 3 Peak" <- w302
    "Filter 4 Peak" <- w301
    "Filter 5 Peak" <- w300
    "Filter 6 Peak" <- w299
    "Filter 7 Peak" <- w298
    n253 = property on="Filter 3 Peak" class="DigNum (strict)"("DisabledEnum"=w273, "Blinking"=w268) -> ()  [unwired: 2 in, 2 out]
    n254 = property on="Filter 4 Peak" class="DigNum (strict)"("DisabledEnum"=w273, "Blinking"=w268) -> ()  [unwired: 2 in, 2 out]
    n255 = property on="Filter 7 Peak" class="DigNum (strict)"("DisabledEnum"=w273, "Blinking"=w268) -> ()  [unwired: 2 in, 2 out]
    n256 = property on="Filter 5 Peak" class="DigNum (strict)"("DisabledEnum"=w273, "Blinking"=w268) -> ()  [unwired: 2 in, 2 out]
    n257 = property on="Filter 6 Peak" class="DigNum (strict)"("DisabledEnum"=w273, "Blinking"=w268) -> ()  [unwired: 2 in, 2 out]
    n258 = property on="Filter 2 Peak" class="DigNum (strict)"("DisabledEnum"=w273, "Blinking"=w268) -> ()  [unwired: 2 in, 2 out]
    n259 = property on="Filter 1 Peak" class="DigNum (strict)"("DisabledEnum"=w273, "Blinking"=w268) -> ()  [unwired: 2 in, 2 out]
    n260 = local read "Update Threshold"() -> (w183:bool)
    n261 = call-poly <userlib>:"Data Changed__ogtk.vi"("Boolean"=w183) -> ("Changed"=w184:bool)
    n262 = And(x=w184, y=w183) -> (x .and. y?=w182:bool)
    n263 = case shown="True" w182 {
      frame False {
      }
      frame True {
        n264 = local write "Update Threshold"(FALSE ("Update Threshold")) -> ()
      }
    }
    n265 = Or(x=w186, y=w183) -> (x .or. y?=w185:bool)
    "Sensitivity" <- w211
  }
  n266 = while {
    stop <- w702 stop-if-true
    n267 = case shown="True" "Rate Limiting" {
      frame False {
        n268 = property on="Rearm Trigger" class="Bool (strict)"("DisabledEnum"=T2."Enabled" ("Disabled")) -> ()  [unwired: 2 in, 2 out]
        n269 = property on="One Shot Mode" class="Bool (strict)"("DisabledEnum"=T2."Enabled" ("Disabled")) -> ()  [unwired: 2 in, 2 out]
      }
      frame True {
        n270 = local read "Armed"() -> (w706:bool)
        n271 = Get Date/Time In Seconds() -> (seconds since 1Jan1904=w705:timestamp)
        n272 = property on="Rearm Trigger" class="Bool (strict)"("DisabledEnum"=T2."Disabled and Grayed Out" ("Disabled")) -> ()  [unwired: 2 in, 2 out]
        n273 = case shown="False" w706 {
          tunnel: [w713 FALSE] -> w710
          tunnel: w705 -> [w712 _]
          frame False {
            n274 = flat-sequence {
              tunnel: w712 -> [w714]
              tunnel: [w714] -> w711
              tunnel: [TRUE] -> w713
              tunnel: w711 -> [w720]
              frame #0 {
                n275 = Multiply(x="Min. Time\nBetween Shots (s)", y=1000.0) -> (x*y=w717:dbl)
                n276 = Round Toward +Infinity(x=w717) -> (ceil(x): smallest int >= x=w715:dbl)
                n277 = Wait (ms)(milliseconds to wait=w715) -> ()  [unwired: 1 out]
              }
              frame #1 {
                n278 = Get Date/Time In Seconds() -> (seconds since 1Jan1904=w721:timestamp)
                n279 = Subtract(x=w721, y=w720) -> (x-y=→"Time Betwee Shots":dbl)
              }
            }
          }
          frame True {
          }
        }
        n280 = property on="One Shot Mode" class="Bool (strict)"("DisabledEnum"=T2."Disabled and Grayed Out" ("Disabled"), "Value"=TRUE ("One Shot Mode")) -> ()  [unwired: 2 in, 2 out]
        n281 = local write "Rearm Trigger"(w710) -> ()
      }
    }
    n282 = property on="stopping" class="Bool (strict)"() -> ("Value"=w702:bool)  [unwired: 2 in, 2 out]
  }
  n283 = call "connect out.vi"("error in (no error)"=w39, "connection reference"=w41) -> ()  [unwired: 9 in, 1 out]
  n284 = xnode "Close FPGA VI Reference"("FPGA VI Reference In"=w65, "error in"=w64) -> ("error out"=w67:errorcluster)
  n285 = call <vilib>:"General Error Handler.vi"("error in (no error)"=w67) -> ()  [unwired: 10 in, 5 out]
